vi "FPGA_compute-next-bus-point.vi"(8 "channel actual":u16, 11 "increase value":bool) -> (1 "next point":u16)   [LabVIEW 2013]
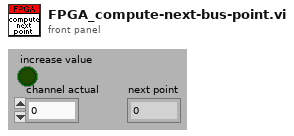
[diagram p1: front panel]
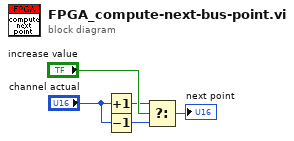
[diagram p0: block diagram]
diagram:
  n1 = Increment(x="channel actual") -> (x+1=w3:u16)
  n2 = Decrement(x="channel actual") -> (x-1=w2:u16)
  n3 = Select(t=w3, s="increase value", f=w2) -> (s? t:f=→"next point":u16)
